vi "BLE_Initialize.vi"(11 "error in (no error)":errorcluster) -> (4 ".NET Refnum out":refnum<k24>, 15 "error out":errorcluster)   [LabVIEW 2020]
uses:
  C:/Users/bharathi.t/Downloads/Bluetooth - Copy/Bluetooth/BLE/BLELib.dll
  BLELib.dll
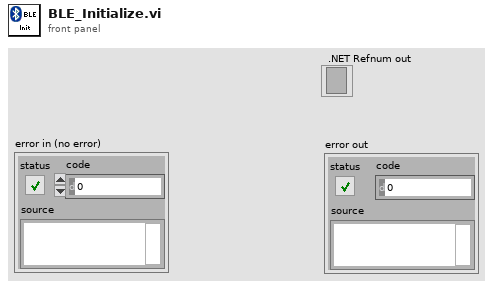
[diagram p1: front panel]
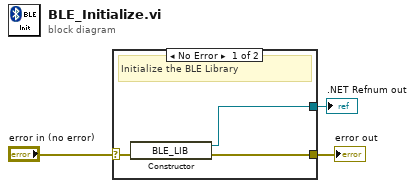
[diagram p0: block diagram]
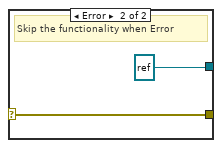
[diagram p2: hidden frame]
diagram:
  n1 = case shown="No Error" "error in (no error)" {
    selector: "error in (no error)" -> [w6 w8]
    tunnel: [w5 w8] -> w2
    tunnel: [w4 refnum<k24> refnum (".NET Refnum out")] -> w1
    frame No Error {
      # "Initialize the BLE Library"
      n2 = constructor class="BLE_LIB"(error in=w6) -> (reference out=w4:refnum<k24>, error out=w5:errorcluster)  [unwired: 2 in, 1 out]
    }
    frame Error {
      # "Skip the functionality when Error"
    }
  }
  "error out" <- w2
  ".NET Refnum out" <- w1
